vi "SCAO-4bArnaud.vi"() -> ()   [LabVIEW 2009]
uses:
  <vilib>/Platform/TimedLoop/XDataNode/XDataNode.xnode
  <vilib>/Platform/TimedLoop/XDataNode/loadlvalarms.vi
  <vilib>/Platform/TimedLoop/XDataNode/timing_clust.ctl
  <vilib>/Platform/TimedLoop/XDataNode/nitl_modes.ctl
  <vilib>/Platform/TimedLoop/XDataNode/wakeup.ctl
  Instance          19 15Saved   SCAO-4b .vi
  Instance          12 15Saved   SCAO-4b .vi
  Instance          16 15Saved   SCAO-4b .vi
  Instance          11 15Saved   SCAO-4b .vi
  Instance          13 15Saved   SCAO-4b .vi
  Instance          15 15Saved   SCAO-4b .vi
  Instance          14 15Saved   SCAO-4b .vi
  Instance           1 15Saved   SCAO-4b .vi
  Instance          17 15Saved   SCAO-4b .vi
  <vilib>/Platform/TimedLoop/XDataNode/XDNodeRunTimeDep.lvlib
panel:
  out "Itération Boucle":i32
  in  "Période":i64
  in  "Température Mesurée":dbl
  out "Durée écoulée":dbl
  in  "Durée imposée":dbl
  out "Time has Elapsed":bool caption="Le temps est écoulé"
  out "Appliqué":bool
  in  "Température imposée":dbl
  out "°C":dbl(knob) caption="données" scale=0.0..100.0
  out "Mesuré < imposé (-1)":bool
  in  "Imposé (-1)":dbl
  out "°C/m2":dbl(knob) scale=-5.0..5.0
  out "220 Volts":bool
  out "Mesuré < imposé":bool
  out "> 55°C":bool
  in  "Imposé":dbl
  out "°C/m":dbl(knob) scale=-5.0..5.0
  in  "ON/OFF":bool
  out "temps actuel":timestamp format="%<>T"
  # "Système de Cuisson Assisté par Ordinateur (SCAO)"
  # "SCAO"
  # "Rouge : VRAI\nVert : FAUX"
  # "Table de cuisson"
  # "Température de cuisson"
  # "Gradient thermique"
  # "Durée de cuisson"
  # "Gradient thermique (-1)"
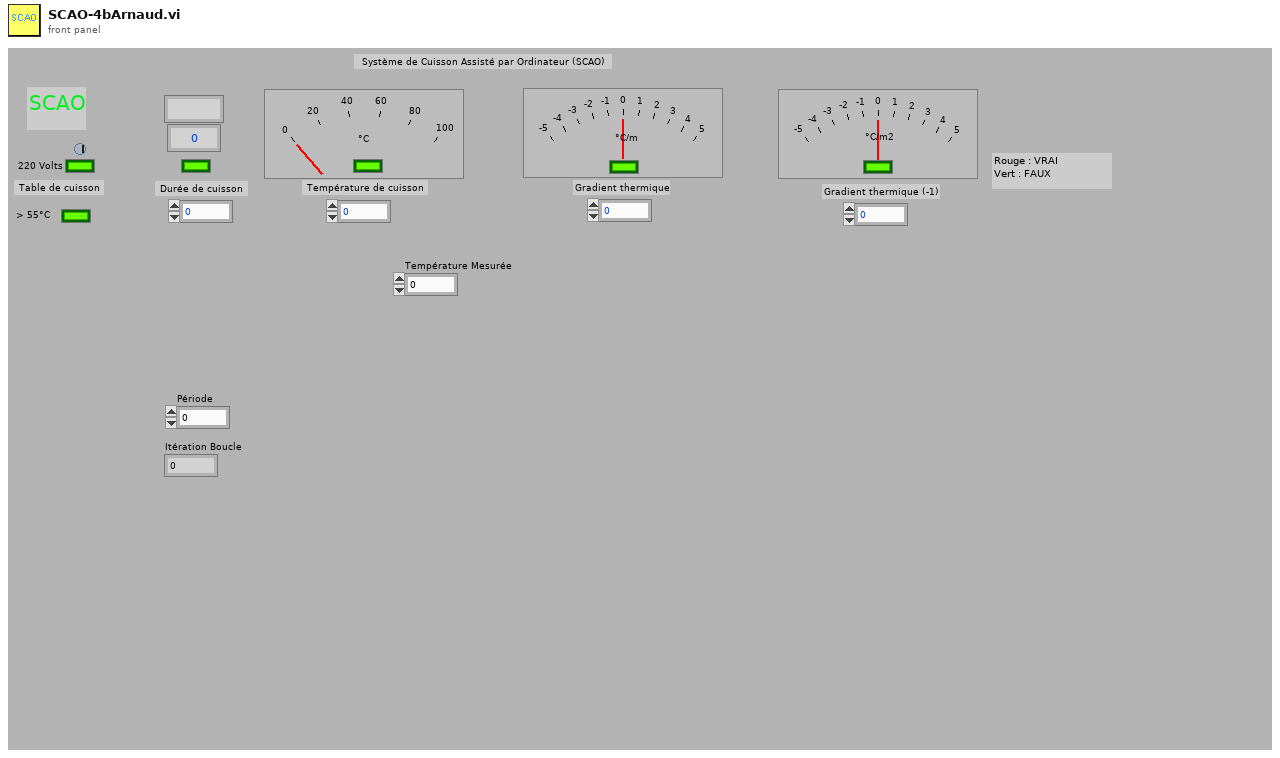
[diagram p1: front panel]
types:
  T1 = enum16{"open", "replace", "create", "open or create", "replace or create", "replace or create with confirmation"}
  T2 = typedef "XDNodeRunTimeDep.lvlib/timing_clust.ctl" = cluster{"Expected End [f-1]":u64, "Actual End [f-1]":u64, "Finished Late? [f-1]":bool, "Expected End [i-1]":u64, "Actual End [i-1]":u64, "Finished Late? [i-1]":bool, "Expected Start [i]":u64, "Actual Start [i]":u64, "Expected Start [f]":u64, "Actual Start [f]":u64, "Source Name":string, "Structure Name":string, "Period":i64, "Deadline":i64, "Offset":i64, "Start":i64, "Priority":i32, "Timeout":i32, "Mode":T3, "Wakeup Reason":T4, "Error":errorcluster, "Source Type":string, "Secondary Source Type":string, "Global End Time":u64, "Global Start Time":u64, "Frame Duration":u64, "Iteration Duration":u64, "Assigned CPU":i32, "I/O Scan Engine Mode":u32}
  T3 = typedef "XDNodeRunTimeDep.lvlib/nitl_modes.ctl" = enum32{"No Change", "Process missed periods, maintain original phase", "Discard missed periods, maintain original phase", "Process missed periods, ignore original phase", "Discard missed periods, ignore original phase"}
  T4 = typedef "XDNodeRunTimeDep.lvlib/wakeup.ctl" = enum32{"Normal", "Aborted", "Asynchronous wakeup", "Timing source error", "Timed loop error", "Timeout"}
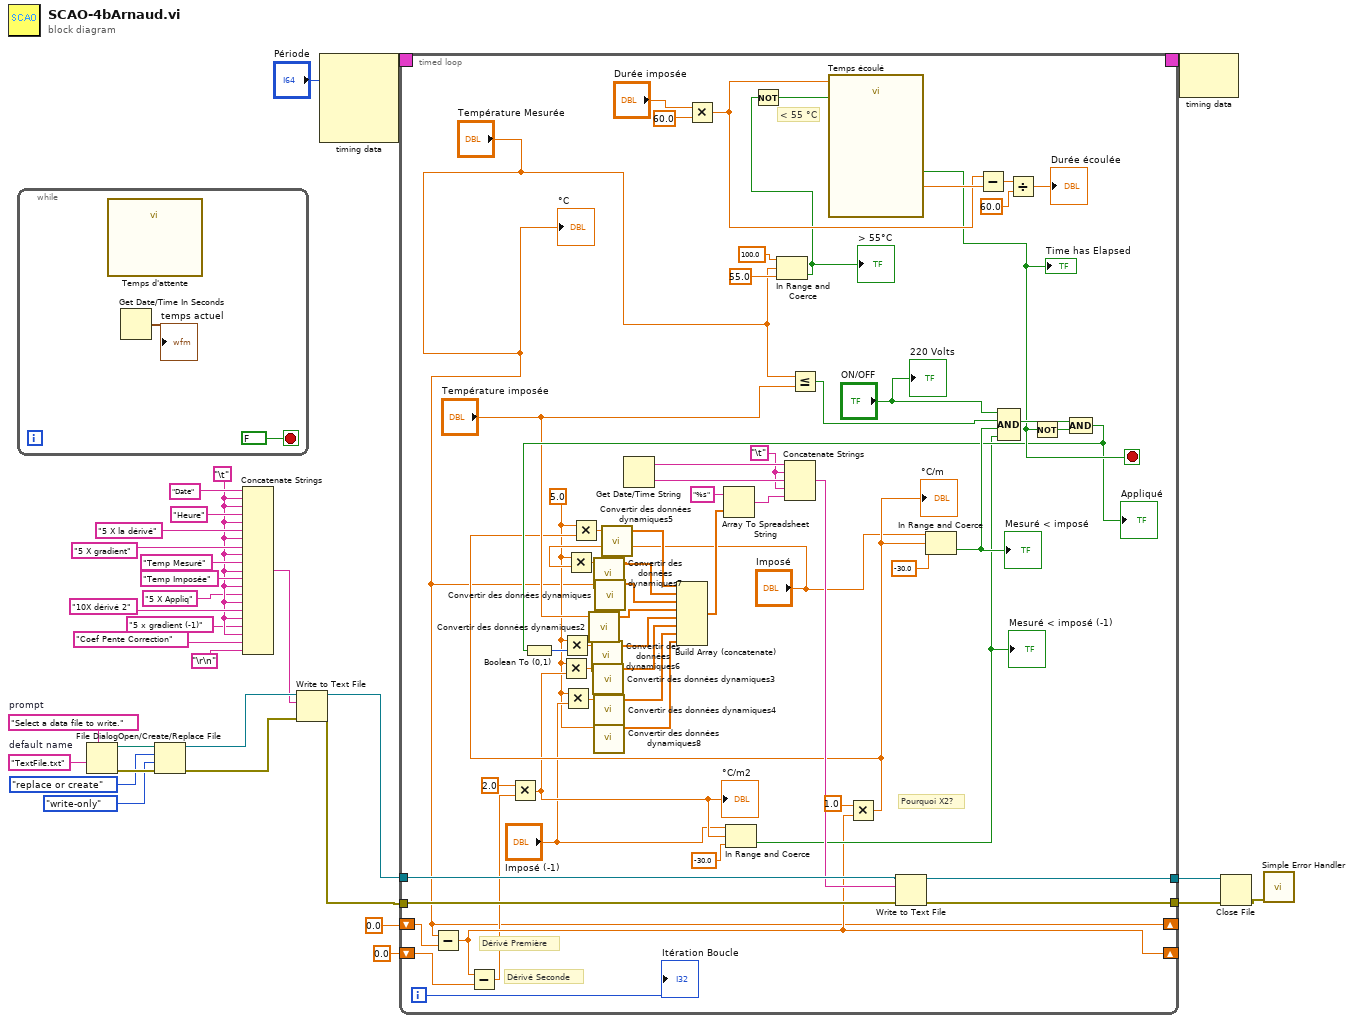
[diagram p0: block diagram]
diagram:
  w4 = "\t" ("Tab")
  w28 = "TextFile.txt"  # default name
  w27 = "Select a data file to write."  # prompt
  n1 = while {
    stop <- FALSE stop-if-true
    n2 = call "Temps d'attente"() -> ()  [unwired: 11 in, 1 out]
    n3 = Get Date/Time In Seconds() -> (seconds since 1Jan1904=→"temps actuel":timestamp)
  }
  n4 = File Dialog(7:w27, 9:w28) -> (0:w26:errorcluster, 3:w29:path)  [unwired: 5 in, 2 out]
  n5 = Open/Create/Replace File(file path (use dialog)=w29, error in=w26, operation (0:open)=T1."replace or create", access (0:read/write)=enum16{"read/write", "read-only", "write-only"}."write-only") -> (refnum out=w17:refnum<file>, error out=w16:errorcluster)  [unwired: 2 in, 1 out]
  n6 = Concatenate Strings("Date" ("chaîne"), w4, w4, "Heure" ("chaîne"), w4, "5 X la dérivé" ("chaîne"), w4, "5 X gradient" ("chaîne"), w4, "Temp Mesuré" ("chaîne"), w4, "Temp Imposée" ("chaîne"), w4, "5 X Appliq" ("chaîne"), w4, "10X dérivé 2" ("chaîne"), w4, "5 x gradient (-1)" ("chaîne"), w4, "Coef Pente Correction" ("chaîne"), "\r\n") -> (w9:string)
  n7 = Write to Text File(file (use dialog)=w17, text=w9, error in=w16) -> (refnum out=w15:refnum<file>, error out=w14:errorcluster)  [unwired: 1 in, 1 out]
  n8 = node-c288("Période") -> (w31:T2)  [unwired: 3 in]
  n9 = timed-loop {
    timing-out: [_] -> w30
    timing: w31 -> [_]
    tunnel: w15 -> [w93]
    tunnel: w14 -> [w92]
    tunnel: [w91] -> w22
    tunnel: [w78] -> w21
    shift-right: ["Température Mesurée"] -> _
    shift-left: 0.0 ("data") -> [w83]
    shift-right: [w52] -> _
    shift-left: 0.0 -> [w65]
    i -> [w35]
    stop <- w69 stop-if-true
    w37 = 5.0 ("x")
    w87 = "\t" ("Tab")
    # "Dérivé Première"
    # "< 55 °C"
    # "Dérivé Seconde"
    # "Pourquoi X2?"
    n10 = Subtract(x="Température Mesurée", y=w83) -> (x-y=w52:dbl)
    n11 = Subtract(x=w52, y=w65) -> (x-y=w50:dbl)
    n12 = Multiply(x=2.0, y=w50) -> (x*y=w43:dbl)
    "°C/m2" <- w43
    n13 = Multiply(x=w37, y=w43) -> (x*y=w44:dbl)
    n14 = Multiply(x=w37, y="Imposé (-1)") -> (x*y=w42:dbl)
    n15 = Multiply(x=w37, y="Imposé") -> (x*y=w46:dbl)
    n16 = call "Convertir des données dynamiques2"("Dynamic Data Type"="Température imposée") -> ("Array"=w61:dbl[])  [unwired: 3 in]
    n17 = call "Convertir des données dynamiques3"("Dynamic Data Type"=w44) -> ("Array"=w58:dbl[])  [unwired: 3 in]
    n18 = call "Convertir des données dynamiques7"("Dynamic Data Type"=w46) -> ("Array"=w59:dbl[])  [unwired: 3 in]
    n19 = call "Convertir des données dynamiques4"("Dynamic Data Type"=w42) -> ("Array"=w57:dbl[])  [unwired: 3 in]
    n20 = call "Convertir des données dynamiques8"("Dynamic Data Type"=w37) -> ("Array"=w38:dbl[])  [unwired: 3 in]
    n21 = call "Convertir des données dynamiques"("Dynamic Data Type"="Température Mesurée") -> ("Array"=w60:dbl[])  [unwired: 3 in]
    n22 = Get Date/Time String() -> (date string=w90:string, time string=w89:string)  [unwired: 3 in]
    n23 = Multiply(x="Durée imposée", y=60.0) -> (x*y=w73:dbl)
    n24 = In Range and Coerce(upper limit="Imposé (-1)", x=w43, lower limit=-30.0 ("limite inférieure")) -> (In Range?=w63:bool)  [unwired: 1 out]
    "Mesuré < imposé (-1)" <- w63
    n25 = In Range and Coerce(upper limit=100.0 ("limite supérieure"), x="Température Mesurée", lower limit=55.0 ("limite inférieure")) -> (In Range?=w56:bool)  [unwired: 1 out]
    "> 55°C" <- w56
    n26 = Not(x=w56) -> (.not. x?=w70:bool)
    n27 = Less Or Equal?(x="Température Mesurée", y="Température imposée") -> (x <= y?=w80:bool)
    n28 = call "Temps écoulé"("Time Target (s)"=w73, "Reset"=w70) -> ("Elapsed Time (s)"=w74:dbl, "Time has Elapsed"=w69:bool)  [unwired: 10 in, 6 out]
    "Time has Elapsed" <- w69
    n29 = Multiply(x=1.0, y=w52) -> (x*y=w47:dbl)
    "°C/m" <- w47
    n30 = Multiply(x=w37, y=w47) -> (x*y=w48:dbl)
    n31 = call "Convertir des données dynamiques5"("Dynamic Data Type"=w48) -> ("Array"=w84:dbl[])  [unwired: 3 in]
    n32 = In Range and Coerce(upper limit="Imposé", x=w47, lower limit=-30.0 ("limite inférieure")) -> (In Range?=w68:bool)  [unwired: 1 out]
    "Mesuré < imposé" <- w68
    n33 = Subtract(x=w73, y=w74) -> (x-y=w72:dbl)
    n34 = Compound Arithmetic op=AND("ON/OFF", w80, w68, w63) -> (w79:bool)
    n35 = Divide(x=w72, y=60.0) -> (x/y=→"Durée écoulée":dbl)
    n36 = Not(x=w69) -> (.not. x?=w81:bool)
    n37 = Compound Arithmetic op=AND(w79, w81) -> (w66:bool)
    "Appliqué" <- w66
    n38 = Boolean To (0,1)(Boolean=w66) -> (0, 1=w39:i16)
    n39 = Multiply(x=w37, y=w39) -> (x*y=w40:dbl)
    n40 = call "Convertir des données dynamiques6"("Dynamic Data Type"=w40) -> ("Array"=w62:dbl[])  [unwired: 3 in]
    n41 = Build Array (concatenate)(w84, w59, w60, w61, w62, w58, w57, w38) -> (w86:dbl[])
    n42 = Array To Spreadsheet String(array=w86, 3:"%s" ("chaîne de format")) -> (spreadsheet string=w85:string)  [unwired: 1 in]
    n43 = Concatenate Strings(w90, w87, w89, w87, w85) -> (w88:string)
    n44 = Write to Text File(file (use dialog)=w93, text=w88, error in=w92) -> (refnum out=w91:refnum<file>, error out=w78:errorcluster)  [unwired: 1 in, 1 out]
    "220 Volts" <- "ON/OFF"
    "°C" <- "Température Mesurée"
    "Itération Boucle" <- w35
  }
  n45 = node-c288(w30) -> ()  [unwired: 1 out]
  n46 = Close File(refnum=w22, error in=w21) -> (error out=w23:errorcluster)  [unwired: 1 out]
  n47 = call <vilib>:"Simple Error Handler.vi"("error in (no error)"=w23) -> ()  [unwired: 4 in, 5 out]
